vi "Read Write Config.vi"(0 "Config File":path, 2 "Read?":bool, 7 "Cluster In":T2, 11 "Error In":errorcluster) -> (8 "Cluster Out":T2, 15 "Error Out":errorcluster)   [LabVIEW 2013]
uses:
  TypeDef/StandConfigCluster.ctl
  <vilib>/Utility/config.llb/Write Key (String).vi
  <vilib>/Utility/config.llb/Write Key (Double).vi
  <vilib>/Utility/config.llb/Write Key (Boolean).vi
  <vilib>/Utility/config.llb/Write Key (I32).vi
  <vilib>/Utility/config.llb/Read Key (String).vi
  <vilib>/Utility/config.llb/Read Key (Double).vi
  <vilib>/Utility/config.llb/Read Key (Boolean).vi
  <vilib>/Utility/config.llb/Read Key (I32).vi
  <vilib>/Utility/config.llb/NI_LVConfig.lvlib
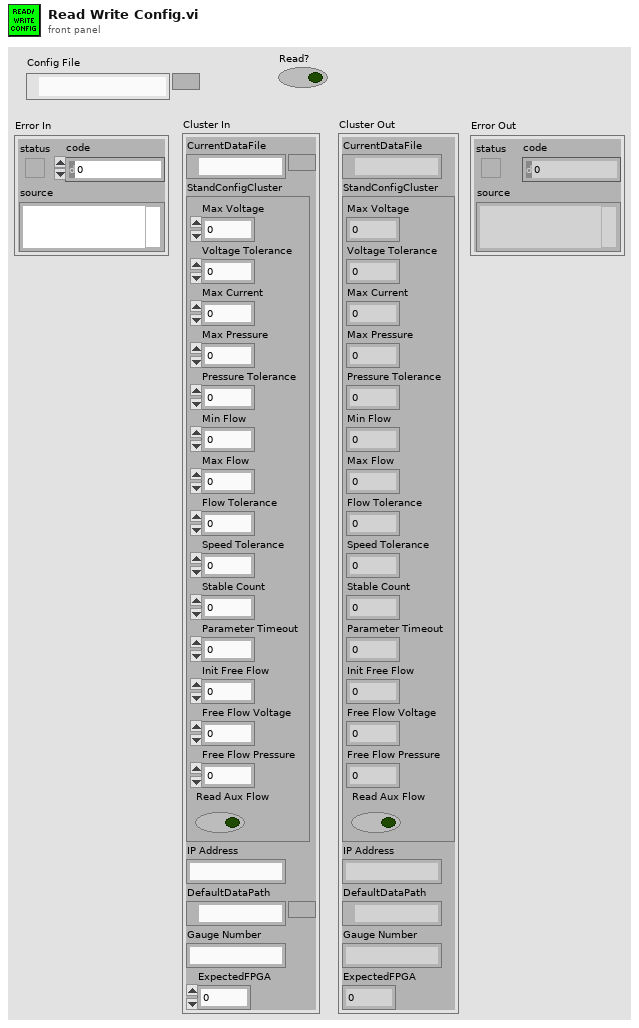
[diagram p1: front panel]
types:
  T1 = typedef "StandConfigCluster.ctl" = cluster{"Max Voltage":dbl, "Voltage Tolerance":dbl, "Max Current":dbl, "Max Pressure":dbl, "Pressure Tolerance":dbl, "Min Flow":dbl, "Max Flow":dbl, "Flow Tolerance":dbl, "Speed Tolerance":dbl, "Stable Count":dbl, "Parameter Timeout":dbl, "Init Free Flow":dbl, "Free Flow Voltage":dbl, "Free Flow Pressure":dbl, "Read Aux Flow":bool}
  T2 = cluster{"CurrentDataFile":path, "StandConfigCluster":T1, "IP Address":string, "DefaultDataPath":path, "Gauge Number":string, "ExpectedFPGA":i32}
  T3 = enum16{"open", "replace", "create", "open or create", "replace or create", "replace or create with confirmation"}
  T4 = typedef "NI_LVConfig.lvlib/Config Data RefNum.ctl" = refnum<k1>
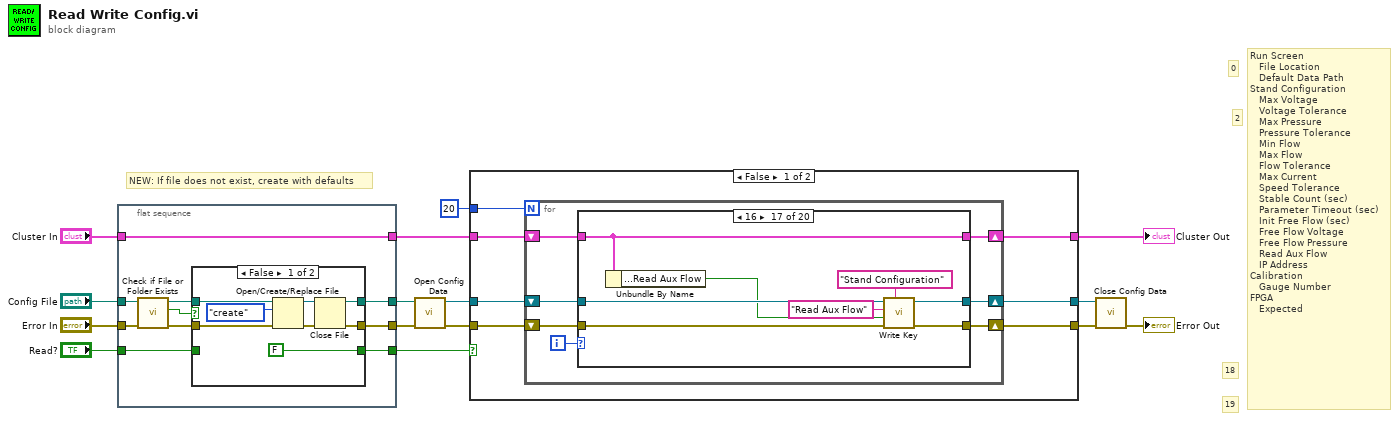
[diagram p0: block diagram]
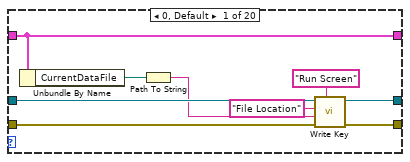
[diagram p3: hidden frame]
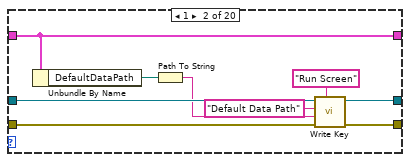
[diagram p4: hidden frame]
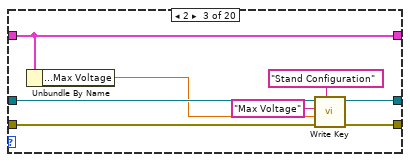
[diagram p5: hidden frame]
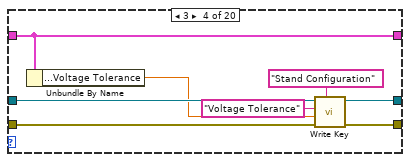
[diagram p6: hidden frame]
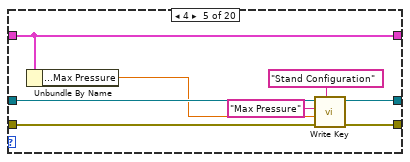
[diagram p7: hidden frame]
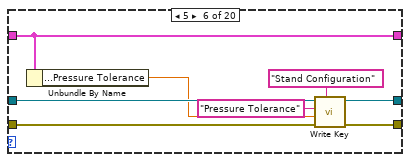
[diagram p8: hidden frame]
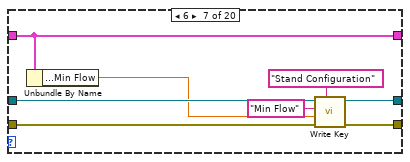
[diagram p9: hidden frame]
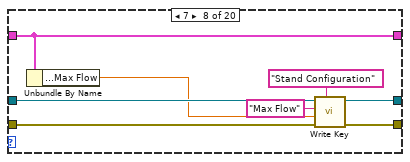
[diagram p10: hidden frame]
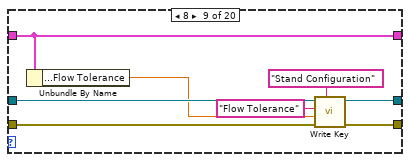
[diagram p11: hidden frame]
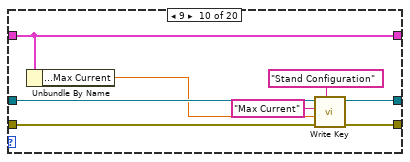
[diagram p12: hidden frame]
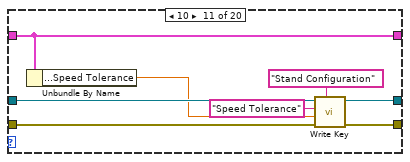
[diagram p13: hidden frame]
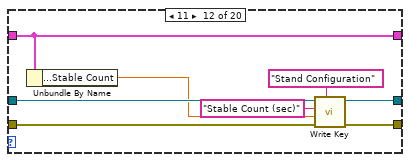
[diagram p14: hidden frame]
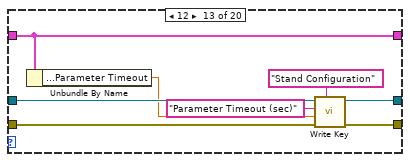
[diagram p15: hidden frame]
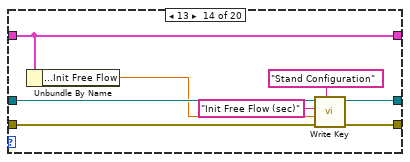
[diagram p16: hidden frame]
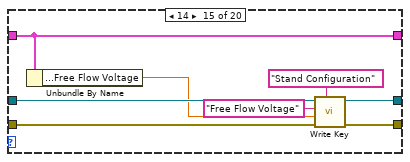
[diagram p17: hidden frame]
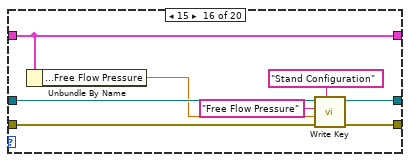
[diagram p18: hidden frame]
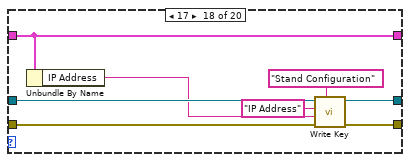
[diagram p19: hidden frame]
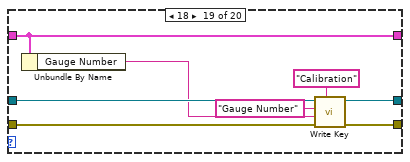
[diagram p20: hidden frame]
diagram:
  # "18"
  # "19"
  # "2"
  # "0"
  # "NEW: If file does not exist, create with defaults"
  # "Run Screen\n   File Location\n   Default Data Path\nStand Configuration\n   Max Voltage\n   Voltage Tolerance\n   Max Pressure\n   Pressure Tolerance\n   Min Flow\n   Max Flow\n   Flow Tolerance\n   Max Current\n   Speed Tolerance\n   Stable Count (sec)\n   Parameter Timeout (sec)\n   Init Free Flow (sec)\n   Free Flow Voltage\n   Free Flow Pressure\n   Read Aux Flow\n   IP Address\nCalibration\n   Gauge Number\nFPGA\n   Expected"
  n1 = flat-sequence {
    tunnel: "Cluster In" -> [w25]
    tunnel: "Config File" -> [w24]
    tunnel: "Error In" -> [w23]
    tunnel: "Read?" -> [w17]
    tunnel: [w25] -> w7
    tunnel: [w19] -> w6
    tunnel: [w18] -> w5
    tunnel: [w16] -> w4
    frame #0 {
      n2 = call <vilib>:"Check if File or Folder Exists.vi"("error in (no error)"=w23, "path"=w24) -> ("error out"=w21:errorcluster, "file or folder exists?"=w22:bool, "dup path"=w20:path)  [unwired: 7 in]
      n3 = case shown="False" w22 {
        tunnel: [w28 w36] -> w18
        tunnel: w21 -> [w31 w36]
        tunnel: [w27 w35] -> w19
        tunnel: w20 -> [w32 w35]
        tunnel: [FALSE w34] -> w16
        tunnel: w17 -> [_ w34]
        frame False {
          n4 = Open/Create/Replace File(file path (use dialog)=w32, error in=w31, operation (0:open)=T3."create") -> (refnum out=w26:refnum<file>, error out=w29:errorcluster)  [unwired: 3 in, 1 out]
          n5 = Close File(refnum=w26, error in=w29) -> (path=w27:path, error out=w28:errorcluster)
        }
        frame True {
        }
      }
    }
  }
  n6 = call <vilib>:"Open Config Data.vi"("error in (no error)"=w5, "configuration file path"=w6) -> ("error out"=w14:errorcluster, "refnum"=w15:T4)  [unwired: 7 in, 1 out]
  n7 = case shown="False" w4 {
    tunnel: w15 -> [w43 w219]
    tunnel: w14 -> [w42 w218]
    tunnel: [w41 w217] -> w13
    tunnel: [w40 w216] -> w12
    tunnel: w7 -> [w39 w215]
    tunnel: [w38 w214] -> w1
    tunnel: 20 -> [w37 w213]
    frame False {
      n8 = for {
        N: w37 -> [_]
        shift-right: [w48] -> w41
        shift-left: w43 -> [w50]
        shift-right: [w47] -> w40
        shift-left: w42 -> [w49]
        shift-right: [w44] -> w38
        shift-left: w39 -> [w45]
        i -> [w46]
        n9 = case shown="16" w46 {
          tunnel: w50 -> [w59 w68 w76 w84 w92 w100 w108 w116 w124 w132 w140 w148 w156 w164 w172 w180 w188 w196 w204 w212]
          tunnel: w49 -> [w58 w67 w75 w83 w91 w99 w107 w115 w123 w131 w139 w147 w155 w163 w171 w179 w187 w195 w203 w211]
          tunnel: [w57 w66 w74 w82 w90 w98 w106 w114 w122 w130 w138 w146 w154 w162 w170 w178 w186 w194 w202 w210] -> w48
          tunnel: [w56 w65 w73 w81 w89 w97 w105 w113 w121 w129 w137 w145 w153 w161 w169 w177 w185 w193 w201 w209] -> w47
          tunnel: w45 -> [w53 w62 w70 w78 w86 w94 w102 w110 w118 w126 w134 w142 w150 w158 w166 w174 w182 w190 w199 w207]
          tunnel: [w53 w62 w70 w78 w86 w94 w102 w110 w118 w126 w134 w142 w150 w158 w166 w174 w182 w190 w199 w207] -> w44
          frame 0, Default {
            n10 = Unbundle By Name(w53) -> ("CurrentDataFile"=w52:path)
            n11 = Path To String(path=w52) -> (string=w51:string)
            n12 = call-poly <vilib>:"Write Key.vi"("section"="Run Screen", "error in (no error)"=w58, "value"=w51, "key"="File Location", "refnum"=w59) -> ("error out"=w56:errorcluster, "refnum out"=w57:T4)  [unwired: 4 in, 1 out]
          }
          frame 1 {
            n13 = Unbundle By Name(w62) -> ("DefaultDataPath"=w61:path)
            n14 = Path To String(path=w61) -> (string=w60:string)
            n15 = call-poly <vilib>:"Write Key.vi"("section"="Run Screen", "error in (no error)"=w67, "value"=w60, "key"="Default Data Path", "refnum"=w68) -> ("error out"=w65:errorcluster, "refnum out"=w66:T4)  [unwired: 4 in, 1 out]
          }
          frame 2 {
            n16 = Unbundle By Name(w70) -> ("StandConfigCluster.Max Voltage"=w69:dbl)
            n17 = call-poly <vilib>:"Write Key.vi"("section"="Stand Configuration", "error in (no error)"=w75, "value"=w69, "key"="Max Voltage", "refnum"=w76) -> ("error out"=w73:errorcluster, "refnum out"=w74:T4)  [unwired: 4 in, 1 out]
          }
          frame 3 {
            n18 = Unbundle By Name(w78) -> ("StandConfigCluster.Voltage Tolerance"=w77:dbl)
            n19 = call-poly <vilib>:"Write Key.vi"("section"="Stand Configuration", "error in (no error)"=w83, "value"=w77, "key"="Voltage Tolerance", "refnum"=w84) -> ("error out"=w81:errorcluster, "refnum out"=w82:T4)  [unwired: 4 in, 1 out]
          }
          frame 4 {
            n20 = Unbundle By Name(w86) -> ("StandConfigCluster.Max Pressure"=w85:dbl)
            n21 = call-poly <vilib>:"Write Key.vi"("section"="Stand Configuration", "error in (no error)"=w91, "value"=w85, "key"="Max Pressure", "refnum"=w92) -> ("error out"=w89:errorcluster, "refnum out"=w90:T4)  [unwired: 4 in, 1 out]
          }
          frame 5 {
            n22 = Unbundle By Name(w94) -> ("StandConfigCluster.Pressure Tolerance"=w93:dbl)
            n23 = call-poly <vilib>:"Write Key.vi"("section"="Stand Configuration", "error in (no error)"=w99, "value"=w93, "key"="Pressure Tolerance", "refnum"=w100) -> ("error out"=w97:errorcluster, "refnum out"=w98:T4)  [unwired: 4 in, 1 out]
          }
          frame 6 {
            n24 = Unbundle By Name(w102) -> ("StandConfigCluster.Min Flow"=w101:dbl)
            n25 = call-poly <vilib>:"Write Key.vi"("section"="Stand Configuration", "error in (no error)"=w107, "value"=w101, "key"="Min Flow", "refnum"=w108) -> ("error out"=w105:errorcluster, "refnum out"=w106:T4)  [unwired: 4 in, 1 out]
          }
          frame 7 {
            n26 = Unbundle By Name(w110) -> ("StandConfigCluster.Max Flow"=w109:dbl)
            n27 = call-poly <vilib>:"Write Key.vi"("section"="Stand Configuration", "error in (no error)"=w115, "value"=w109, "key"="Max Flow", "refnum"=w116) -> ("error out"=w113:errorcluster, "refnum out"=w114:T4)  [unwired: 4 in, 1 out]
          }
          frame 8 {
            n28 = Unbundle By Name(w118) -> ("StandConfigCluster.Flow Tolerance"=w117:dbl)
            n29 = call-poly <vilib>:"Write Key.vi"("section"="Stand Configuration", "error in (no error)"=w123, "value"=w117, "key"="Flow Tolerance", "refnum"=w124) -> ("error out"=w121:errorcluster, "refnum out"=w122:T4)  [unwired: 4 in, 1 out]
          }
          frame 9 {
            n30 = Unbundle By Name(w126) -> ("StandConfigCluster.Max Current"=w125:dbl)
            n31 = call-poly <vilib>:"Write Key.vi"("section"="Stand Configuration", "error in (no error)"=w131, "value"=w125, "key"="Max Current", "refnum"=w132) -> ("error out"=w129:errorcluster, "refnum out"=w130:T4)  [unwired: 4 in, 1 out]
          }
          frame 10 {
            n32 = Unbundle By Name(w134) -> ("StandConfigCluster.Speed Tolerance"=w133:dbl)
            n33 = call-poly <vilib>:"Write Key.vi"("section"="Stand Configuration", "error in (no error)"=w139, "value"=w133, "key"="Speed Tolerance", "refnum"=w140) -> ("error out"=w137:errorcluster, "refnum out"=w138:T4)  [unwired: 4 in, 1 out]
          }
          frame 11 {
            n34 = Unbundle By Name(w142) -> ("StandConfigCluster.Stable Count"=w141:dbl)
            n35 = call-poly <vilib>:"Write Key.vi"("section"="Stand Configuration", "error in (no error)"=w147, "value"=w141, "key"="Stable Count (sec)", "refnum"=w148) -> ("error out"=w145:errorcluster, "refnum out"=w146:T4)  [unwired: 4 in, 1 out]
          }
          frame 12 {
            n36 = Unbundle By Name(w150) -> ("StandConfigCluster.Parameter Timeout"=w149:dbl)
            n37 = call-poly <vilib>:"Write Key.vi"("section"="Stand Configuration", "error in (no error)"=w155, "value"=w149, "key"="Parameter Timeout (sec)", "refnum"=w156) -> ("error out"=w153:errorcluster, "refnum out"=w154:T4)  [unwired: 4 in, 1 out]
          }
          frame 13 {
            n38 = Unbundle By Name(w158) -> ("StandConfigCluster.Init Free Flow"=w157:dbl)
            n39 = call-poly <vilib>:"Write Key.vi"("section"="Stand Configuration", "error in (no error)"=w163, "value"=w157, "key"="Init Free Flow (sec)", "refnum"=w164) -> ("error out"=w161:errorcluster, "refnum out"=w162:T4)  [unwired: 4 in, 1 out]
          }
          frame 14 {
            n40 = Unbundle By Name(w166) -> ("StandConfigCluster.Free Flow Voltage"=w165:dbl)
            n41 = call-poly <vilib>:"Write Key.vi"("section"="Stand Configuration", "error in (no error)"=w171, "value"=w165, "key"="Free Flow Voltage", "refnum"=w172) -> ("error out"=w169:errorcluster, "refnum out"=w170:T4)  [unwired: 4 in, 1 out]
          }
          frame 15 {
            n42 = Unbundle By Name(w174) -> ("StandConfigCluster.Free Flow Pressure"=w173:dbl)
            n43 = call-poly <vilib>:"Write Key.vi"("section"="Stand Configuration", "error in (no error)"=w179, "value"=w173, "key"="Free Flow Pressure", "refnum"=w180) -> ("error out"=w177:errorcluster, "refnum out"=w178:T4)  [unwired: 4 in, 1 out]
          }
          frame 16 {
            n44 = Unbundle By Name(w182) -> ("StandConfigCluster.Read Aux Flow"=w181:bool)
            n45 = call-poly <vilib>:"Write Key.vi"("section"="Stand Configuration", "error in (no error)"=w187, "value"=w181, "key"="Read Aux Flow", "refnum"=w188) -> ("error out"=w185:errorcluster, "refnum out"=w186:T4)  [unwired: 4 in, 1 out]
          }
          frame 17 {
            n46 = Unbundle By Name(w190) -> ("IP Address"=w189:string)
            n47 = call-poly <vilib>:"Write Key.vi"("section"="Stand Configuration", "error in (no error)"=w195, "value"=w189, "key"="IP Address", "refnum"=w196) -> ("error out"=w193:errorcluster, "refnum out"=w194:T4)  [unwired: 4 in, 1 out]
          }
          frame 18 {
            n48 = Unbundle By Name(w199) -> ("Gauge Number"=w197:string)
            n49 = call-poly <vilib>:"Write Key.vi"("section"="Calibration", "error in (no error)"=w203, "value"=w197, "key"="Gauge Number", "refnum"=w204) -> ("error out"=w201:errorcluster, "refnum out"=w202:T4)  [unwired: 4 in, 1 out]
          }
          frame 19 {
            n50 = Unbundle By Name(w207) -> ("ExpectedFPGA"=w205:i32)
            n51 = call-poly <vilib>:"Write Key.vi"("section"="FPGA", "error in (no error)"=w211, "value"=w205, "key"="Expected", "refnum"=w212) -> ("error out"=w209:errorcluster, "refnum out"=w210:T4)  [unwired: 4 in, 1 out]
          }
        }
      }
    }
    frame True {
      n52 = for {
        N: w213 -> [_]
        shift-right: [w224] -> w217
        shift-left: w219 -> [w226]
        shift-right: [w223] -> w216
        shift-left: w218 -> [w225]
        shift-right: [w220] -> w214
        shift-left: w215 -> [w221]
        i -> [w222]
        n53 = case shown="16" w222 {
          tunnel: w226 -> [w236 w246 w255 w264 w273 w282 w291 w300 w309 w318 w327 w336 w345 w354 w363 w372 w381 w390 w399 w408]
          tunnel: w225 -> [w235 w245 w254 w263 w272 w281 w290 w299 w308 w317 w326 w335 w344 w353 w362 w371 w380 w389 w398 w407]
          tunnel: [w234 w244 w253 w262 w271 w280 w289 w298 w307 w316 w325 w334 w343 w352 w361 w370 w379 w388 w397 w406] -> w224
          tunnel: [w233 w243 w252 w261 w270 w279 w288 w297 w306 w315 w324 w333 w342 w351 w360 w369 w378 w387 w396 w405] -> w223
          tunnel: w221 -> [w232 w242 w251 w260 w269 w278 w287 w296 w305 w314 w323 w332 w341 w350 w359 w368 w377 w386 w393 w402]
          tunnel: [w231 w241 w250 w259 w268 w277 w286 w295 w304 w313 w322 w331 w340 w349 w358 w367 w376 w385 w392 w401] -> w220
          frame 0, Default {
            n54 = call-poly <vilib>:"Read Key.vi"("section"="Run Screen", "error in (no error)"=w235, "key"="File Location", "refnum"=w236) -> ("error out"=w233:errorcluster, "value"=w228:string, "refnum out"=w234:T4)  [unwired: 4 in, 1 out]
            n55 = String To Path(string=w228) -> (path=w227:path)
            n56 = Bundle By Name(cluster=w232, "CurrentDataFile"=w227) -> (w231:T2)
          }
          frame 1 {
            n57 = call-poly <vilib>:"Read Key.vi"("section"="Run Screen", "error in (no error)"=w245, "key"="Default Data Path", "refnum"=w246) -> ("error out"=w243:errorcluster, "value"=w238:string, "refnum out"=w244:T4)  [unwired: 4 in, 1 out]
            n58 = String To Path(string=w238) -> (path=w237:path)
            n59 = Bundle By Name(cluster=w242, "DefaultDataPath"=w237) -> (w241:T2)
          }
          frame 2 {
            n60 = call-poly <vilib>:"Read Key.vi"("section"="Stand Configuration", "error in (no error)"=w254, "key"="Max Voltage", "refnum"=w255) -> ("error out"=w252:errorcluster, "value"=w247:dbl, "refnum out"=w253:T4)  [unwired: 4 in, 1 out]
            n61 = Bundle By Name(cluster=w251, "StandConfigCluster.Max Voltage"=w247) -> (w250:T2)
          }
          frame 3 {
            n62 = call-poly <vilib>:"Read Key.vi"("section"="Stand Configuration", "error in (no error)"=w263, "key"="Voltage Tolerance", "refnum"=w264) -> ("error out"=w261:errorcluster, "value"=w256:dbl, "refnum out"=w262:T4)  [unwired: 4 in, 1 out]
            n63 = Bundle By Name(cluster=w260, "StandConfigCluster.Voltage Tolerance"=w256) -> (w259:T2)
          }
          frame 4 {
            n64 = call-poly <vilib>:"Read Key.vi"("section"="Stand Configuration", "error in (no error)"=w272, "key"="Max Pressure", "refnum"=w273) -> ("error out"=w270:errorcluster, "value"=w265:dbl, "refnum out"=w271:T4)  [unwired: 4 in, 1 out]
            n65 = Bundle By Name(cluster=w269, "StandConfigCluster.Max Pressure"=w265) -> (w268:T2)
          }
          frame 5 {
            n66 = call-poly <vilib>:"Read Key.vi"("section"="Stand Configuration", "error in (no error)"=w281, "key"="Pressure Tolerance", "refnum"=w282) -> ("error out"=w279:errorcluster, "value"=w274:dbl, "refnum out"=w280:T4)  [unwired: 4 in, 1 out]
            n67 = Bundle By Name(cluster=w278, "StandConfigCluster.Pressure Tolerance"=w274) -> (w277:T2)
          }
          frame 6 {
            n68 = call-poly <vilib>:"Read Key.vi"("section"="Stand Configuration", "error in (no error)"=w290, "key"="Min Flow", "refnum"=w291) -> ("error out"=w288:errorcluster, "value"=w283:dbl, "refnum out"=w289:T4)  [unwired: 4 in, 1 out]
            n69 = Bundle By Name(cluster=w287, "StandConfigCluster.Min Flow"=w283) -> (w286:T2)
          }
          frame 7 {
            n70 = call-poly <vilib>:"Read Key.vi"("section"="Stand Configuration", "error in (no error)"=w299, "key"="Max Flow", "refnum"=w300) -> ("error out"=w297:errorcluster, "value"=w292:dbl, "refnum out"=w298:T4)  [unwired: 4 in, 1 out]
            n71 = Bundle By Name(cluster=w296, "StandConfigCluster.Max Flow"=w292) -> (w295:T2)
          }
          frame 8 {
            n72 = call-poly <vilib>:"Read Key.vi"("section"="Stand Configuration", "error in (no error)"=w308, "key"="Flow Tolerance", "refnum"=w309) -> ("error out"=w306:errorcluster, "value"=w301:dbl, "refnum out"=w307:T4)  [unwired: 4 in, 1 out]
            n73 = Bundle By Name(cluster=w305, "StandConfigCluster.Flow Tolerance"=w301) -> (w304:T2)
          }
          frame 9 {
            n74 = call-poly <vilib>:"Read Key.vi"("section"="Stand Configuration", "error in (no error)"=w317, "key"="Max Current", "refnum"=w318) -> ("error out"=w315:errorcluster, "value"=w310:dbl, "refnum out"=w316:T4)  [unwired: 4 in, 1 out]
            n75 = Bundle By Name(cluster=w314, "StandConfigCluster.Max Current"=w310) -> (w313:T2)
          }
          frame 10 {
            n76 = call-poly <vilib>:"Read Key.vi"("section"="Stand Configuration", "error in (no error)"=w326, "key"="Speed Tolerance", "refnum"=w327) -> ("error out"=w324:errorcluster, "value"=w319:dbl, "refnum out"=w325:T4)  [unwired: 4 in, 1 out]
            n77 = Bundle By Name(cluster=w323, "StandConfigCluster.Speed Tolerance"=w319) -> (w322:T2)
          }
          frame 11 {
            n78 = call-poly <vilib>:"Read Key.vi"("section"="Stand Configuration", "error in (no error)"=w335, "key"="Stable Count (sec)", "refnum"=w336) -> ("error out"=w333:errorcluster, "value"=w328:dbl, "refnum out"=w334:T4)  [unwired: 4 in, 1 out]
            n79 = Bundle By Name(cluster=w332, "StandConfigCluster.Stable Count"=w328) -> (w331:T2)
          }
          frame 12 {
            n80 = call-poly <vilib>:"Read Key.vi"("section"="Stand Configuration", "error in (no error)"=w344, "key"="Parameter Timeout (sec)", "refnum"=w345) -> ("error out"=w342:errorcluster, "value"=w337:dbl, "refnum out"=w343:T4)  [unwired: 4 in, 1 out]
            n81 = Bundle By Name(cluster=w341, "StandConfigCluster.Parameter Timeout"=w337) -> (w340:T2)
          }
          frame 13 {
            n82 = call-poly <vilib>:"Read Key.vi"("section"="Stand Configuration", "error in (no error)"=w353, "key"="Init Free Flow (sec)", "refnum"=w354) -> ("error out"=w351:errorcluster, "value"=w346:dbl, "refnum out"=w352:T4)  [unwired: 4 in, 1 out]
            n83 = Bundle By Name(cluster=w350, "StandConfigCluster.Init Free Flow"=w346) -> (w349:T2)
          }
          frame 14 {
            n84 = call-poly <vilib>:"Read Key.vi"("section"="Stand Configuration", "error in (no error)"=w362, "key"="Free Flow Voltage", "refnum"=w363) -> ("error out"=w360:errorcluster, "value"=w355:dbl, "refnum out"=w361:T4)  [unwired: 4 in, 1 out]
            n85 = Bundle By Name(cluster=w359, "StandConfigCluster.Free Flow Voltage"=w355) -> (w358:T2)
          }
          frame 15 {
            n86 = call-poly <vilib>:"Read Key.vi"("section"="Stand Configuration", "error in (no error)"=w371, "key"="Free Flow Pressure", "refnum"=w372) -> ("error out"=w369:errorcluster, "value"=w364:dbl, "refnum out"=w370:T4)  [unwired: 4 in, 1 out]
            n87 = Bundle By Name(cluster=w368, "StandConfigCluster.Free Flow Pressure"=w364) -> (w367:T2)
          }
          frame 16 {
            n88 = call-poly <vilib>:"Read Key.vi"("section"="Stand Configuration", "error in (no error)"=w380, "key"="Read Aux Flow", "refnum"=w381) -> ("error out"=w378:errorcluster, "value"=w373:bool, "refnum out"=w379:T4)  [unwired: 4 in, 1 out]
            n89 = Bundle By Name(cluster=w377, "StandConfigCluster.Read Aux Flow"=w373) -> (w376:T2)
          }
          frame 17 {
            n90 = call-poly <vilib>:"Read Key.vi"("section"="Stand Configuration", "error in (no error)"=w389, "key"="IP Address", "refnum"=w390) -> ("error out"=w387:errorcluster, "value"=w382:string, "refnum out"=w388:T4)  [unwired: 4 in, 1 out]
            n91 = Bundle By Name(cluster=w386, "IP Address"=w382) -> (w385:T2)
          }
          frame 18 {
            n92 = call-poly <vilib>:"Read Key.vi"("section"="Calibration", "error in (no error)"=w398, "key"="Gauge Number", "refnum"=w399) -> ("error out"=w396:errorcluster, "value"=w391:string, "refnum out"=w397:T4)  [unwired: 4 in, 1 out]
            n93 = Bundle By Name(cluster=w393, "Gauge Number"=w391) -> (w392:T2)
          }
          frame 19 {
            n94 = call-poly <vilib>:"Read Key.vi"("section"="FPGA", "error in (no error)"=w407, "key"="Expected", "refnum"=w408) -> ("error out"=w405:errorcluster, "value"=w400:i32, "refnum out"=w406:T4)  [unwired: 4 in, 1 out]
            n95 = Bundle By Name(cluster=w402, "ExpectedFPGA"=w400) -> (w401:T2)
          }
        }
      }
    }
  }
  "Cluster Out" <- w1
  n96 = call <vilib>:"Close Config Data.vi"("error in (no error)"=w12, "refnum"=w13) -> ("error out"=→"Error Out":errorcluster)  [unwired: 8 in, 1 out]
